vi "Day05-02_전자레인지 프로젝트.vi"() -> ()   [LabVIEW 2021]
panel:
  out "출력 메시지":string
  out "조리 시간":string
  in  "1분":bool
  in  "30초":bool
  in  "10초":bool
  out "LED":bool
  in  "문 열림":bool
  in  "취소":bool
  in  "조리 시작":bool
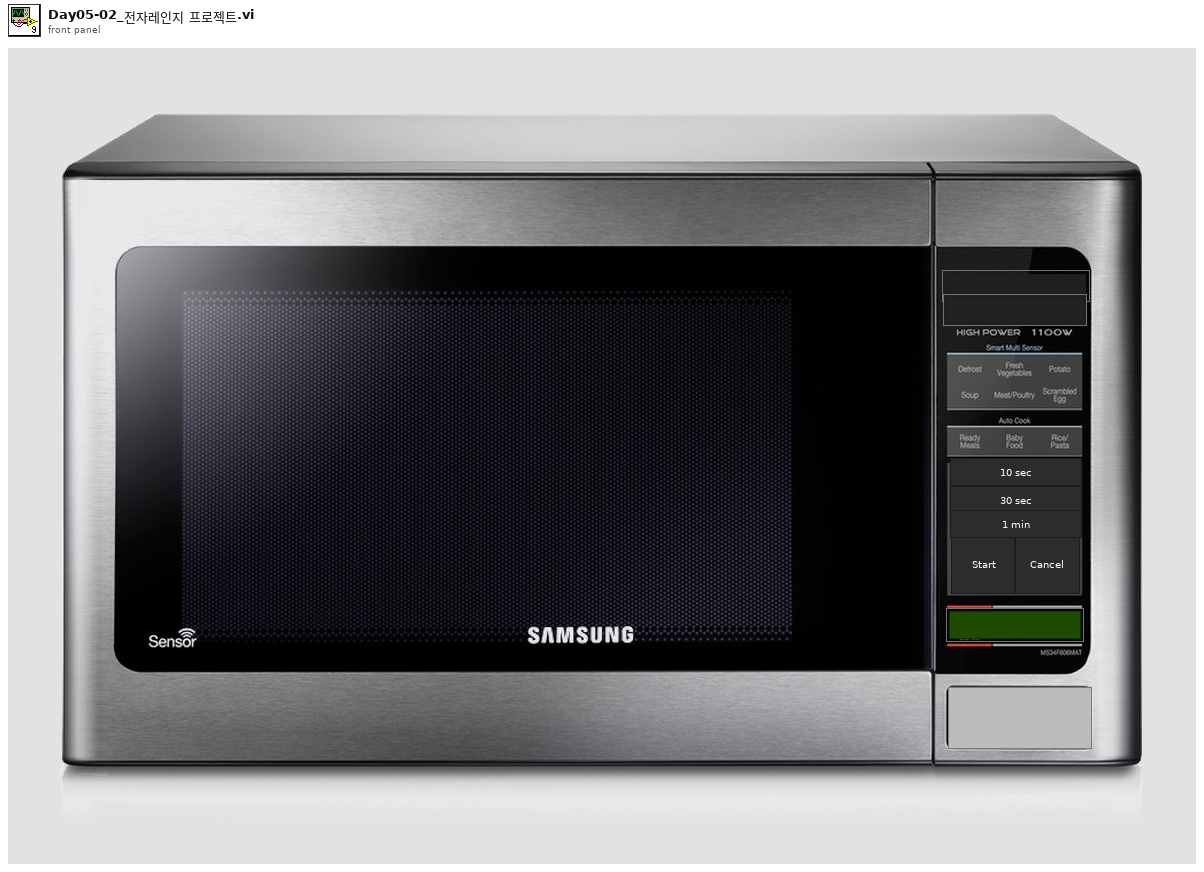
[diagram p1: front panel]
types:
  T1 = cluster{"LED":bool, "조리 시간":string, "출력 메시지":string, "조리시간_1":i32, "pre_tick":i32}
  T2 = typedef "전자레인지 프로젝트 열거형 상수.ctl" = enum16{"초기화", "조리시작", "10초", "30초", "1분", "문 열림", "취소"}
  T3 = enum8{"Enabled", "Disabled", "Disabled and Grayed Out"}
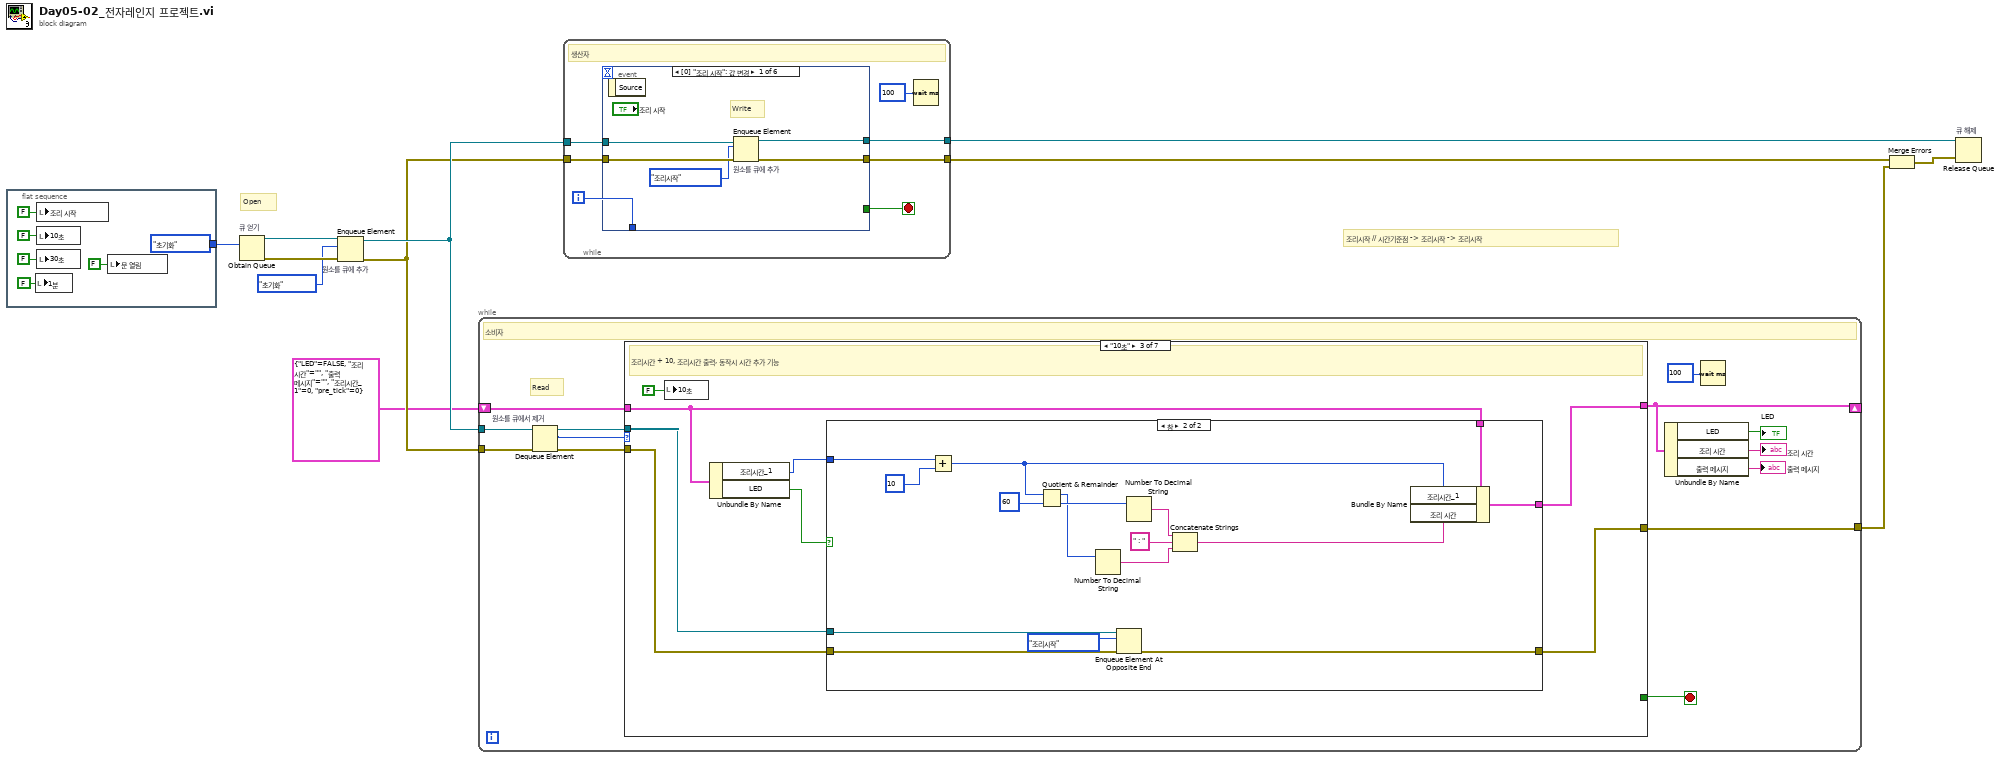
[diagram p0: block diagram]
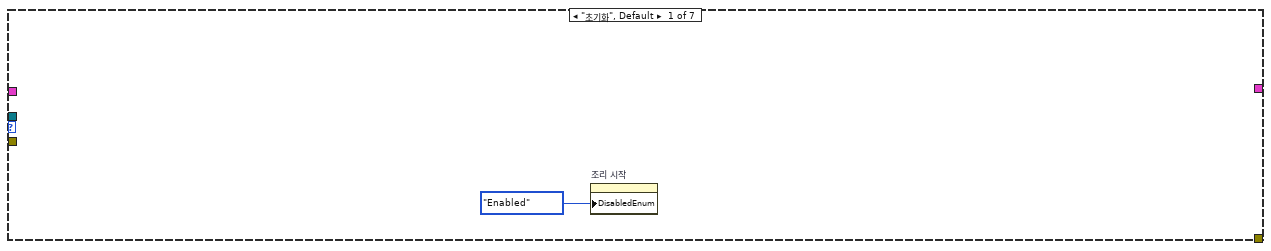
[diagram p2: hidden frame]
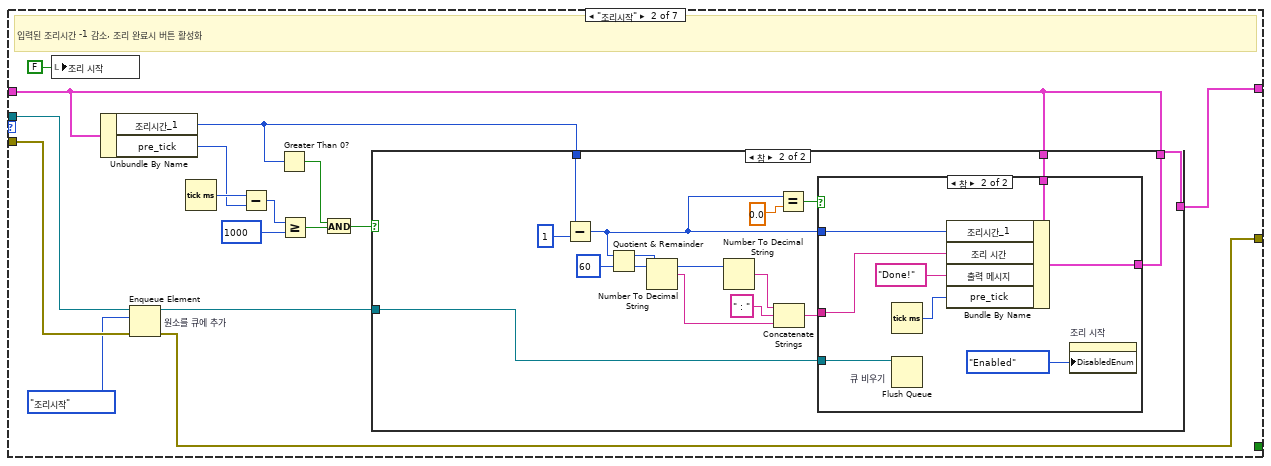
[diagram p3: hidden frame]
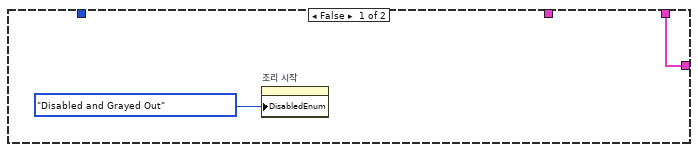
[diagram p4: hidden frame]
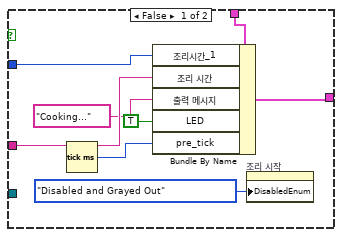
[diagram p5: hidden frame]
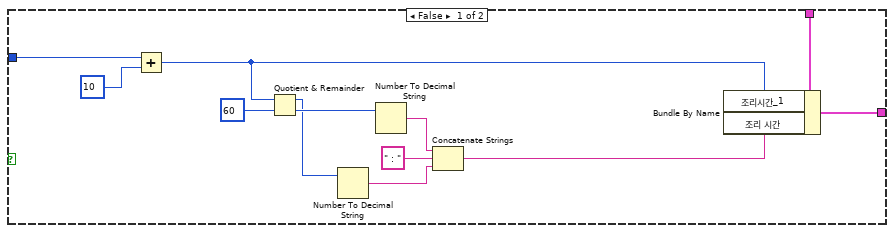
[diagram p6: hidden frame]
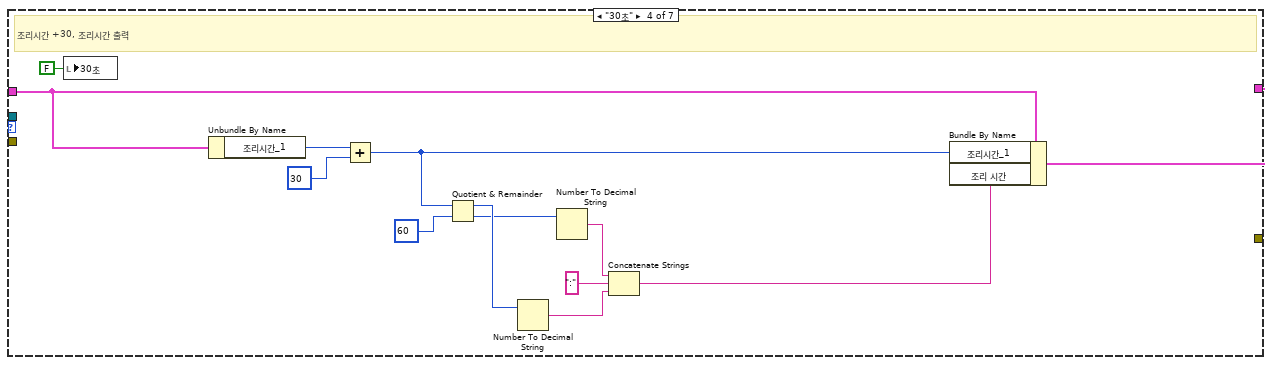
[diagram p7: hidden frame]
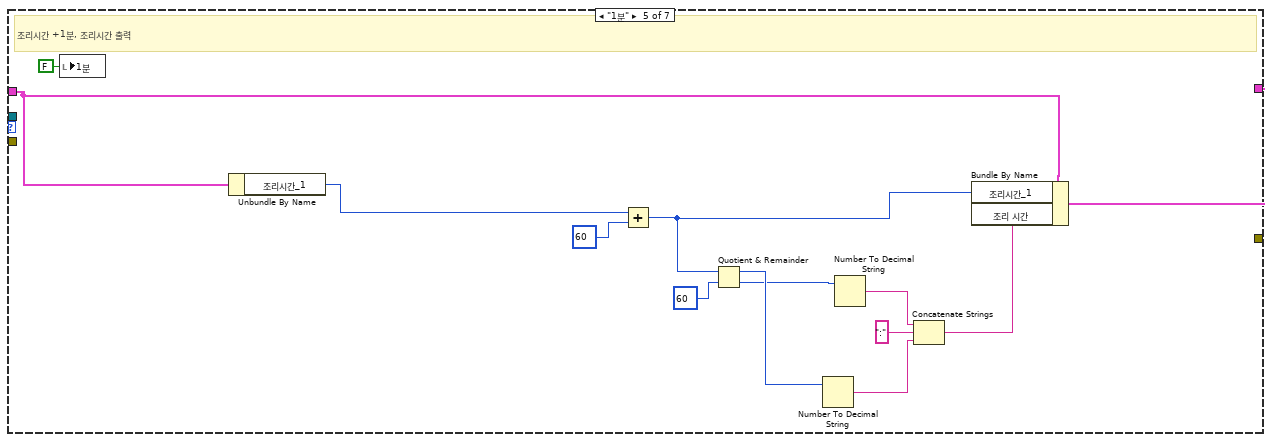
[diagram p8: hidden frame]
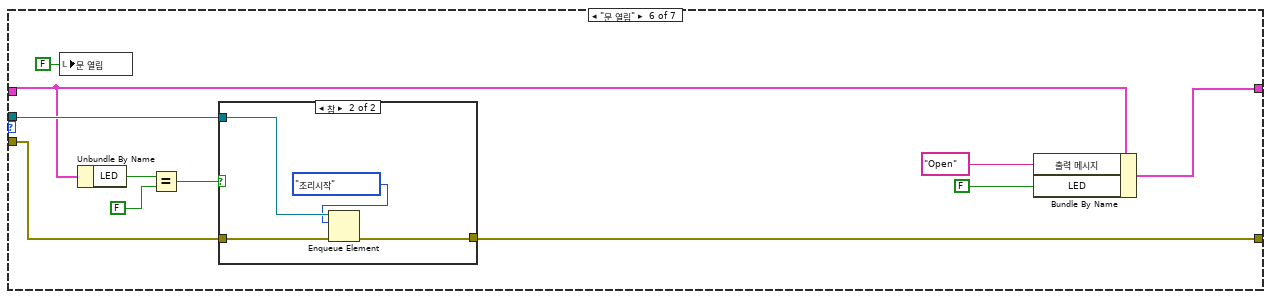
[diagram p9: hidden frame]
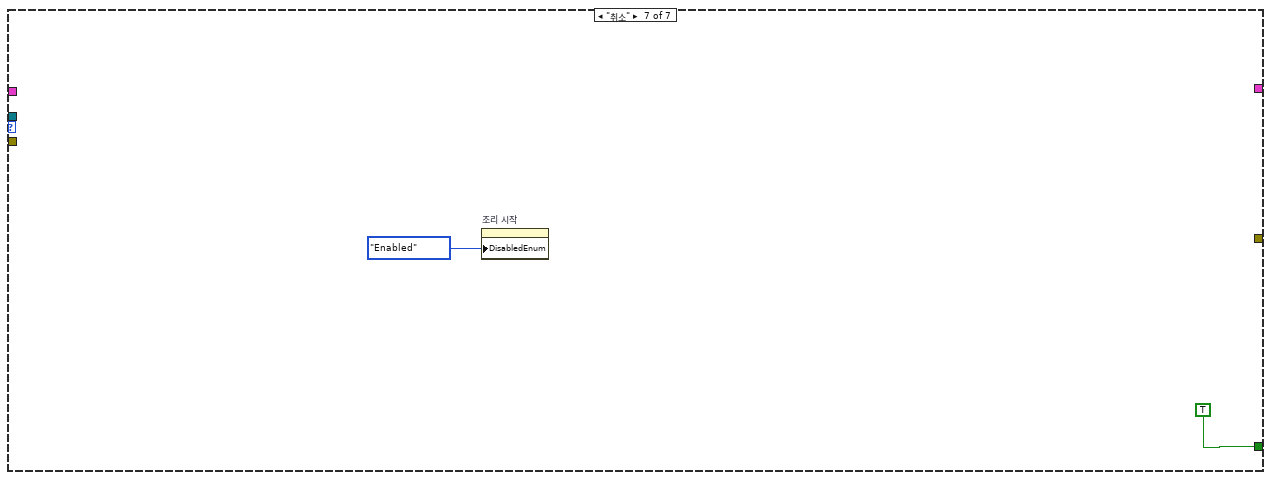
[diagram p11: hidden frame]
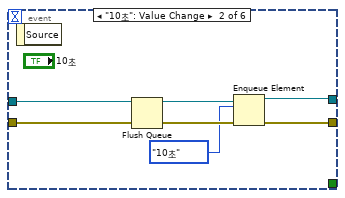
[diagram p12: hidden frame]
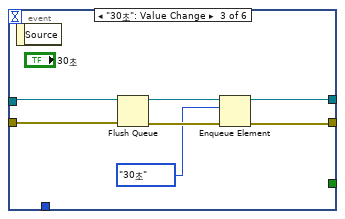
[diagram p13: hidden frame]
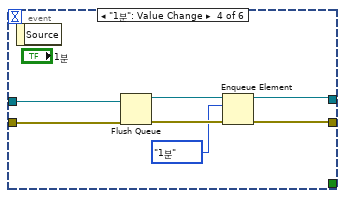
[diagram p14: hidden frame]
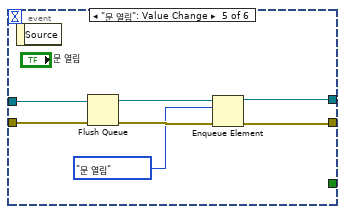
[diagram p15: hidden frame]
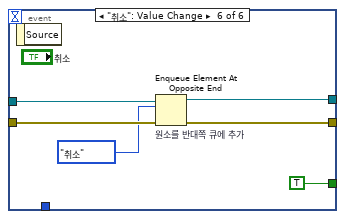
[diagram p16: hidden frame]
diagram:
  # "조리시작 // 시간기준점 -> 조리시작 -> 조리시작"
  # "Open"
  n1 = flat-sequence {
    tunnel: [전자레인지_프로젝트_열거형_상수."초기화"] -> w7
    frame #0 {
      n2 = local write "1분"(FALSE ("1분")) -> ()
      n3 = local write "조리 시작"(FALSE ("조리 시작")) -> ()
      n4 = local write "10초"(FALSE ("10초")) -> ()
      n5 = local write "30초"(FALSE ("30초")) -> ()
      n6 = local write "문 열림"(FALSE ("문 열림")) -> ()
    }
  }
  n7 = Obtain Queue "큐 얻기"(element data type=w7) -> (queue out=w6:refnum<queue>, error out=w4:errorcluster)  [unwired: 4 in, 1 out]
  n8 = Enqueue Element "원소를 큐에 추가"(queue=w6, element=전자레인지_프로젝트_열거형_상수."초기화", error in (no error)=w4) -> (queue out=w5:refnum<queue>, error out=w3:errorcluster)  [unwired: 1 in, 1 out]
  n9 = while {
    tunnel: w5 -> [w30]
    tunnel: w3 -> [w29]
    tunnel: [w26] -> w9
    shift-right: [w22] -> _
    shift-left: T1 {"LED"=FALSE, "조리 시간"="", "출력 메시지"="", "조리시간_1"=0, "pre_tick"=0} -> [w24]
    stop <- w19 stop-if-true
    # "Read"
    # "소비자"
    n10 = Dequeue Element "원소를 큐에서 제거"(queue=w30, error in (no error)=w29) -> (queue out=w28:refnum<queue>, element=w25:T2, error out=w27:errorcluster)  [unwired: 1 in, 1 out]
    n11 = case shown="\"10초\"" w25 {
      tunnel: w28 -> [_ w47 w84 _ _ w148 _]
      tunnel: w27 -> [_ w46 w82 _ _ w147 _]
      tunnel: [_ w45 w83 _ _ w146 _] -> w26
      tunnel: w24 -> [_ w37 w87 w124 w136 w145 _]
      tunnel: [_ w42 w86 w123 w135 w153 _] -> w22
      tunnel: [_ _ _ _ _ _ TRUE] -> w19
      frame "초기화", Default {
        n12 = property on="조리 시작" class="Bool (엄격한)"("DisabledEnum"=T3."Enabled" ("비활성화")) -> ()  [unwired: 2 in, 2 out]
      }
      frame "조리시작" {
        # "입력된 조리시간 -1 감소, 조리 완료시 버튼 활성화"
        n13 = local write "조리 시작"(FALSE ("조리 시작")) -> ()
        n14 = Unbundle By Name(w37) -> ("조리시간_1"=w43:i32, "pre_tick"=w40:i32)
        n15 = Enqueue Element "원소를 큐에 추가"(queue=w47, element=전자레인지_프로젝트_열거형_상수."조리시작" ("원소"), error in (no error)=w46) -> (queue out=w32:refnum<queue>, error out=w45:errorcluster)  [unwired: 1 in, 1 out]
        n16 = Tick Count (ms)() -> (millisecond timer value=w41:u32)
        n17 = Subtract(x=w41, y=w40) -> (x-y=w35:u32)
        n18 = Greater Than 0?(x=w43) -> (x > 0?=w36:bool)
        n19 = Greater Or Equal?(x=w35, y=u32 1000) -> (x >= y?=w34:bool)
        n20 = And(x=w36, y=w34) -> (x .and. y?=w38:bool)
        n21 = case shown="참" w38 {
          tunnel: w37 -> [_ w53]
          tunnel: w43 -> [_ w52]
          tunnel: [w49 w51] -> w42
          tunnel: w37 -> [w49 _]
          tunnel: w32 -> [_ w50]
          frame False {
            n22 = property on="조리 시작" class="Bool (엄격한)"("DisabledEnum"=T3."Disabled and Grayed Out" ("비활성화")) -> ()  [unwired: 2 in, 2 out]
          }
          frame True {
            n23 = Subtract(x=w52, y=1) -> (x-y=w55:i32)
            n24 = Quotient & Remainder(x=w55, y=60) -> (x-y*floor(x/y)=w61:i32, floor(x/y)=w60:i32)
            n25 = Number To Decimal String(number=w61) -> (decimal integer string=w58:string)  [unwired: 1 in]
            n26 = Number To Decimal String(number=w60) -> (decimal integer string=w59:string)  [unwired: 1 in]
            n27 = Concatenate Strings(w59, " : " ("문자열"), w58) -> (w54:string)
            n28 = Equal?(x=w55, y=0.0) -> (x = y?=w56:bool)
            n29 = case shown="참" w56 {
              tunnel: w55 -> [w72 w80]
              tunnel: w54 -> [w71 w79]
              tunnel: [w68 w78] -> w51
              tunnel: w53 -> [w69 w76]
              tunnel: w50 -> [_ w73]
              frame False {
                n30 = Tick Count (ms)() -> (millisecond timer value=w66:u32)
                n31 = Bundle By Name(cluster=w69, "조리시간_1"=w72, "조리 시간"=w71, "출력 메시지"="Cooking...", "LED"=TRUE, "pre_tick"=w66) -> (w68:T1)
                n32 = property on="조리 시작" class="Bool (엄격한)"("DisabledEnum"=T3."Disabled and Grayed Out" ("비활성화")) -> ()  [unwired: 2 in, 2 out]
              }
              frame True {
                n33 = Tick Count (ms)() -> (millisecond timer value=w75:u32)
                n34 = Flush Queue "큐 비우기"(queue=w73) -> ()  [unwired: 1 in, 3 out]
                n35 = Bundle By Name(cluster=w76, "조리시간_1"=w80, "조리 시간"=w79, "출력 메시지"="Done!", "pre_tick"=w75) -> (w78:T1)
                n36 = property on="조리 시작" class="Bool (엄격한)"("DisabledEnum"=T3."Enabled" ("비활성화")) -> ()  [unwired: 2 in, 2 out]
              }
            }
          }
        }
      }
      frame "10초" {
        # "조리시간 + 10, 조리시간 출력, 동작시 시간 추가 기능"
        n37 = local write "10초"(FALSE ("10초")) -> ()
        n38 = Unbundle By Name(w87) -> ("조리시간_1"=w88:i32, "LED"=w85:bool)
        n39 = case shown="참" w85 {
          tunnel: w88 -> [w91 w116]
          tunnel: w87 -> [w90 w115]
          tunnel: [w89 w114] -> w86
          tunnel: w84 -> [_ w106]
          tunnel: w82 -> [_ w105]
          tunnel: [_ w104] -> w83
          frame False {
            n40 = Add(x=w91, y=10) -> (x+y=w95:i32)
            n41 = Quotient & Remainder(x=w95, y=60) -> (x-y*floor(x/y)=w92:i32, floor(x/y)=w94:i32)
            n42 = Number To Decimal String(number=w92) -> (decimal integer string=w98:string)  [unwired: 1 in]
            n43 = Number To Decimal String(number=w94) -> (decimal integer string=w99:string)  [unwired: 1 in]
            n44 = Concatenate Strings(w99, " : " ("문자열"), w98) -> (w97:string)
            n45 = Bundle By Name(cluster=w90, "조리시간_1"=w95, "조리 시간"=w97) -> (w89:T1)
          }
          frame True {
            n46 = Add(x=w116, y=10) -> (x+y=w108:i32)
            n47 = Quotient & Remainder(x=w108, y=60) -> (x-y*floor(x/y)=w101:i32, floor(x/y)=w107:i32)
            n48 = Number To Decimal String(number=w101) -> (decimal integer string=w111:string)  [unwired: 1 in]
            n49 = Enqueue Element At Opposite End(queue=w106, element=전자레인지_프로젝트_열거형_상수."조리시작" ("원소"), error in (no error)=w105) -> (error out=w104:errorcluster)  [unwired: 1 in, 2 out]
            n50 = Number To Decimal String(number=w107) -> (decimal integer string=w112:string)  [unwired: 1 in]
            n51 = Concatenate Strings(w112, " : " ("문자열"), w111) -> (w110:string)
            n52 = Bundle By Name(cluster=w115, "조리시간_1"=w108, "조리 시간"=w110) -> (w114:T1)
          }
        }
      }
      frame "30초" {
        # "조리시간 +30, 조리시간 출력"
        n53 = local write "30초"(FALSE ("30초")) -> ()
        n54 = Unbundle By Name(w124) -> ("조리시간_1"=w129:i32)
        n55 = Add(x=w129, y=30) -> (x+y=w121:i32)
        n56 = Quotient & Remainder(x=w121, y=60) -> (x-y*floor(x/y)=w120:i32, floor(x/y)=w119:i32)
        n57 = Number To Decimal String(number=w120) -> (decimal integer string=w126:string)  [unwired: 1 in]
        n58 = Number To Decimal String(number=w119) -> (decimal integer string=w127:string)  [unwired: 1 in]
        n59 = Concatenate Strings(w127, ":" ("문자열"), w126) -> (w125:string)
        n60 = Bundle By Name(cluster=w124, "조리시간_1"=w121, "조리 시간"=w125) -> (w123:T1)
      }
      frame "1분" {
        # "조리시간 +1분, 조리시간 출력"
        n61 = local write "1분"(FALSE ("1분")) -> ()
        n62 = Unbundle By Name(w136) -> ("조리시간_1"=w142:i32)
        n63 = Add(x=w142, y=60) -> (x+y=w133:i32)
        n64 = Quotient & Remainder(x=w133, y=60) -> (x-y*floor(x/y)=w132:i32, floor(x/y)=w131:i32)
        n65 = Number To Decimal String(number=w132) -> (decimal integer string=w138:string)  [unwired: 1 in]
        n66 = Number To Decimal String(number=w131) -> (decimal integer string=w139:string)  [unwired: 1 in]
        n67 = Concatenate Strings(w139, ":" ("문자열"), w138) -> (w137:string)
        n68 = Bundle By Name(cluster=w136, "조리시간_1"=w133, "조리 시간"=w137) -> (w135:T1)
      }
      frame "문 열림" {
        n69 = local write "문 열림"(FALSE ("문 열림")) -> ()
        n70 = Unbundle By Name(w145) -> ("LED"=w150:bool)
        n71 = Equal?(x=w150, y=FALSE) -> (x = y?=w149:bool)
        n72 = case shown="참" w149 {
          tunnel: w148 -> [_ w157]
          tunnel: w147 -> [_ w156]
          tunnel: [_ w155] -> w146
          frame False {
          }
          frame True {
            n73 = Enqueue Element(queue=w157, element=전자레인지_프로젝트_열거형_상수."조리시작" ("원소"), error in (no error)=w156) -> (error out=w155:errorcluster)  [unwired: 1 in, 2 out]
          }
        }
        n74 = Bundle By Name(cluster=w145, "출력 메시지"="Open", "LED"=FALSE) -> (w153:T1)
      }
      frame "취소" {
        n75 = property on="조리 시작" class="Bool (엄격한)"("DisabledEnum"=T3."Enabled" ("비활성화")) -> ()  [unwired: 2 in, 2 out]
      }
    }
    n76 = Unbundle By Name(w22) -> ("LED"=→"LED":bool, "조리 시간"=→"조리 시간":string, "출력 메시지"=→"출력 메시지":string)
    n77 = Wait (ms)(milliseconds to wait=u32 100 ("대기 시간 (ms)")) -> ()  [unwired: 1 out]
  }
  n78 = while {
    tunnel: w5 -> [w166]
    tunnel: w3 -> [w165]
    tunnel: [w163] -> w11
    tunnel: [w162] -> w10
    i -> [w164]
    stop <- w160 stop-if-true
    # "생산자"
    n79 = event shown="[0] \"조리 시작\": 값 변경" {
      selector: _ -> [_ _ _ _ _ _]
      dyn-events: _ -> [_ _ _ _ _ _]
      timeout: _ -> [_ _ _ _ _ _]
      tunnel: w166 -> [w171 w178 w182 w189 w199 w205]
      tunnel: w165 -> [w170 w177 w181 w188 w198 w203]
      tunnel: w164 -> [_ _ _ _ _ _]
      tunnel: [w169 w174 w180 w187 w195 w204] -> w163
      tunnel: [w168 w173 w179 w186 w194 w202] -> w162
      tunnel: [_ _ _ _ _ TRUE] -> w160
      event "조리 시작": Value Change {
        # "Write"
        n80 = event-data() -> ()  [unwired: 1 in, 1 out]
        n81 = Enqueue Element "원소를 큐에 추가"(queue=w171, element=전자레인지_프로젝트_열거형_상수."조리시작", error in (no error)=w170) -> (queue out=w169:refnum<queue>, error out=w168:errorcluster)  [unwired: 1 in, 1 out]
      }
      event "10초": Value Change {
        n82 = event-data() -> ()  [unwired: 1 in, 1 out]
        n83 = Flush Queue(queue=w178, error in (no error)=w177) -> (queue out=w175:refnum<queue>, error out=w176:errorcluster)  [unwired: 1 out]
        n84 = Enqueue Element(queue=w175, element=전자레인지_프로젝트_열거형_상수."10초", error in (no error)=w176) -> (queue out=w174:refnum<queue>, error out=w173:errorcluster)  [unwired: 1 in, 1 out]
      }
      event "30초": Value Change {
        n85 = event-data() -> ()  [unwired: 1 in, 1 out]
        n86 = Flush Queue(queue=w182, error in (no error)=w181) -> (queue out=w184:refnum<queue>, error out=w185:errorcluster)  [unwired: 1 out]
        n87 = Enqueue Element(queue=w184, element=전자레인지_프로젝트_열거형_상수."30초", error in (no error)=w185) -> (queue out=w180:refnum<queue>, error out=w179:errorcluster)  [unwired: 1 in, 1 out]
      }
      event "1분": Value Change {
        n88 = event-data() -> ()  [unwired: 1 in, 1 out]
        n89 = Flush Queue(queue=w189, error in (no error)=w188) -> (queue out=w191:refnum<queue>, error out=w192:errorcluster)  [unwired: 1 out]
        n90 = Enqueue Element(queue=w191, element=전자레인지_프로젝트_열거형_상수."1분", error in (no error)=w192) -> (queue out=w187:refnum<queue>, error out=w186:errorcluster)  [unwired: 1 in, 1 out]
      }
      event "문 열림": Value Change {
        n91 = event-data() -> ()  [unwired: 1 in, 1 out]
        n92 = Flush Queue(queue=w199, error in (no error)=w198) -> (queue out=w197:refnum<queue>, error out=w196:errorcluster)  [unwired: 1 out]
        n93 = Enqueue Element(queue=w197, element=전자레인지_프로젝트_열거형_상수."문 열림", error in (no error)=w196) -> (queue out=w195:refnum<queue>, error out=w194:errorcluster)  [unwired: 1 in, 1 out]
      }
      event "취소": Value Change {
        n94 = event-data() -> ()  [unwired: 1 in, 1 out]
        n95 = Enqueue Element At Opposite End "원소를 반대쪽 큐에 추가"(queue=w205, element=전자레인지_프로젝트_열거형_상수."취소", error in (no error)=w203) -> (queue out=w204:refnum<queue>, error out=w202:errorcluster)  [unwired: 1 in, 1 out]
      }
    }
    n96 = Wait (ms)(milliseconds to wait=u32 100 ("대기 시간 (ms)")) -> ()  [unwired: 1 out]
  }
  n97 = Merge Errors(w10, w9) -> (w8:errorcluster)
  n98 = Release Queue "큐 해제"(queue=w11, error in (no error)=w8) -> ()  [unwired: 1 in, 3 out]
